vi "Axis-To-SIAM-direkt.vi"(7 "Extra Information":u32=255, 8 "error in (no error)":errorcluster, 10 "Position":dbl(slide)=1021459.0 scale=0.0..1000.0, 11 "Axis-Ring":T4=16777217 items=["255Axis"=16777217, "1-Axis"=17825793, "2-Axis"=18874369, "3-Axis"=19922945, "4-Axis"=20971521, "5-Axis"=22020097, "6-Axis"=23068673, "7-Axis"=24117249, "LED365"=2684354561, "LED385"=2685403137, "LED440"=2686451713, "LED470"=2687500289, "LED510"=2688548865, "LED540"=2689597441, "LED590"=2690646017, "LED640"=2691694593, "DurchR"=2701131777, "DurchG"=2702180353, "DurchB"=2703228929, "AF"=2704277505, "Laser0"=2717908993, "Laser1"=2718957569, "Laser2"=2720006145, "Laser3"=2721054721, "Servo0"=67108865, "Servo1"=68157441, "Servo2"=69206017, "Servo3"=70254593, "0-TMSI"=100663361, "1-TMSI"=101711937, "x-tmsi"=102760513, "y-tmsi"=103809089, "z-tmsi"=104857665, "orca1"=503316481, "orca2"=503316482, "orca3"=503316483, "orca4"=503316484, ""=0]) -> (0 "error out":errorcluster, 3 "Direct Commands":T6(array[cluster]) {"command" format="%x" items=["end_no_ticket"=4027514895, "end_ticket"=4027518991, "NoOp"=4026531840, "Read ticks"=4026535936, "Read ticks to var"=4026535938, "Read IP"=4043313152, "Read IP into var"=4043313154, "Set IP from var"=4043309059, "Set IP from var, relative"=4043313155, "branchRel_if_equal"=4043374849, "decrement_branchRel_if_equal"=4043374945, "decrement_branchRel_if_greaterequal"=4043375201, "decrement_branchRel_if_greaterequal_withTicket"=4043379297, "decrement_branchRel_if_smaller"=4043375457, "increment_branchRel_if_smaller"=4043375473, "readVar"=4060090368, "writeVar"=4060086273, "copyVar0_from_var1"=4060086275, "math_addToVariable"=4076863488, "math_addVToVariable"=4076863489, "math_subToVariable"=4076863490, "math_subVToVariable"=4076863491, "math_multToVariable"=4076863492, "math_multvToVariable"=4076863493, "math_divideToVariable"=4076863494, "math_divideVToVariable"=4076863495, "math_modToVariable"=4076863496, "math_modVToVariable"=4076863497, "logic_and"=4093640704, "logic_or"=4093640706, "logic_xor"=4093640708, "bitshift"=4093640712, "I2C-write"=335544337, "I2C-read"=335548433, "Cam-SPI-write"=3254779905, "UART0-VC-Baud-write"=469958673, "UART0-VC-Baud-read"=469962768, "UART0-VC-write"=469762065, "UART0-VC-write-Var"=469762067, "UART0-VC-read-availabe-bytes-to-var"=470355970, "UART0-VC-read-availabe-bytes"=470355984, "UART0-VC-read-skip-bytes"=469831681, "UART0-VC-read"=469766160, "UART0-VC-read-Var"=469766162, "UART1-TSM-Baud-write"=486735889, "UART1-TSM-Baud-read"=486739984, "UART1-TSM-write"=486539281, "UART1-TSM-write-Var"=486539283, "UART1-TSM-read-availabe-bytes-to-var"=487133186, "UART1-TSM-read-availabe-bytes"=487133200, "UART1-TSM-read-skip-bytes"=486604801, "UART1-TSM-read-skip-bytes"=486608897, "UART1-TSM-read"=486543376, "UART1-TSM-read-Var"=486543378, "UART2-Laser-Baud-write"=503513105, "UART2-Baud-read"=503517200, "UART2-write"=503316497, "UART2-write-Var"=503316499, "UART2-read-availabe-bytes-to-var"=503910402, "UART2-read-availabe-bytes"=503910416, "UART2-read-skip-bytes"=503386113, "UART2-read"=503320592, "UART2-read-Var"=503320594, "UART3-Baud-write"=520290321, "UART3-Baud-read"=520294416, "UART3-write"=520093713, "UART3-write-Var"=520093715, "UART3-read-availabe-bytes-to-var"=520687618, "UART3-read-availabe-bytes"=520687632, "UART3-read-skip-bytes"=520163329, "UART3-read"=520097808, "UART3-read-Var"=520097810, "IO-read_bank0"=3489665024, "IO-write_bank0"=3489660929, "IO-read_bank1"=3506442240, "IO-write_bank1"=3506438145, "DA0-0_LED365"=2684354561, "DA0-1_LED385"=2685403137, "DA0-2_LED440"=2686451713, "DA0-3_LED470"=2687500289, "DA0-4_LED510"=2688548865, "DA0-5_LED550"=2689597441, "DA0-6_LED590"=2690646017, "DA0-7_LED640"=2691694593, "DA1-0_LED-R"=2701131777, "DA1-1_LED-G"=2702180353, "DA1-2_LED-B"=2703228929, "DA1-3_LED-AF"=2704277505, "DA1-4"=2705326081, "DA1-5"=2706374657, "DA1-6"=2707423233, "DA1-7"=2708471809, "DA2-Laser0"=2717908993, "DA2-Laser1"=2718957569, "DA2-Laser2"=2720006145, "DA2-Laser3"=2721054721, "DA2-Laser4"=2722103297, "Analog-read_AD0-0"=2818576384, "Analog-read-store_AD0-0"=2818572290, "AF-Register-transfer r/w"=2835349505, "AF-Register-read"=2835353600, "AF-Register-read-to-var"=2835353602, "AF-Transfer-from-var"=2835349507, "IO-delay_bank0"=3489923073, "IO-delay_bank0_fromVar"=3489923075, "read_cam_clock"=3289124864, "store_cam_clock"=3289120770, "read_cam_phase"=3289190400, "store_cam_phase"=3289186306, "store_cam_phase-t"=3289190402, "r_cam1_NHS"=3254980608, "w_cam1_NHS"=3254976513, "r_cam1_NVS"=3255046144, "w_cam1_NVS"=3255042049, "r_cam1_npx"=3255111680, "w_cam1_npx"=3255107585, "r_cam1_npy"=3255177216, "w_cam1_npy"=3255173121, "r_cam1_xhswait"=3255439360, "w_cam1_xhswait"=3255435265, "r_cam1_xvs_wait"=3255504896, "w_cam1_xvs_wait"=3255500801, "r_cam1_framcounter"=3255570432, "r_cam1_line"=3255635968, "r_cam1_xhs-counter"=3255701504, "r_cam2_NHS"=3271757824, "w_cam2_NHS"=3271753729, "r_cam2_NVS"=3271823360, "w_cam2_NVS"=3271819265, "r_cam2_npx"=3271888896, "w_cam2_npx"=3271884801, "r_cam2_npy"=3271954432, "w_cam2_npy"=3271950337, "r_cam2_xvs_wait"=3272282112, "w_cam2_xvs_wait"=3272278017, "r_cam2_framcounter"=3272347648, "r_cam2_line"=3272413184, "r_cam2_xhs-counter"=3272478720, "start TMSI"=102694919, "set_1Galvo"=101712113, "set_x-Galvo"=102760689, "set_y-Galvo"=103809265, "set_z-Fokus"=104857841, "set_1Galvo_position-only"=101711937, "set_x-Galvo_position-only"=102760513, "set_y-Galvo_position-only"=103809089, "set_z-Fokus_position-only"=104857665, "set_x-Galvo_position-only_ticket"=102764609, "set_y-Galvo_position-only_ticket"=103813185, "set_z-Fokus_position-only_ticket"=104861761, "set_1Galvo_relativ-only"=101712001, "set_x-Galvo_relativ-only"=102760577, "set_y-Galvo_relativ-only"=103809153, "set_z-Fokus_relativ-only"=104857729, "set_1Galvo_speed-only"=101711905, "set_x-Galvo_speed-only"=102760481, "set_y-Galvo_speed-only"=103809057, "set_z-Fokus_speed-only"=104857633, "set_1Galvo_acc-only"=101711889, "set_x-Galvo_acc-only"=102760465, "set_y-Galvo_acc-only"=103809041, "set_z-Fokus_acc-only"=104857617, "read_1Galvo_ticket"=101716032, "read_x-Galvo_ticket"=102764608, "read_y-Galvo_ticket"=103813184, "read_z-Focus_ticket"=104861760, "x-Galvo_pos_fromVar"=102760515, "y-Galvo_pos_fromVar"=103809091, "z-Focus_pos_fromVar"=104857667, "Servo0"=67108865, "Servo0-enable"=68091911, "Servo0-disable"=68091919, "Servo1"=68157441, "Servo1-enable"=69140487, "Servo1-disable"=69140495, "Servo2-enable"=70189063, "Servo2"=69206017, "Servo3-enable"=71237639, "Servo3"=70254593, "x-ssi-init"=202309639, "x-ssi-disable"=202309647, "x-ssi-Bits"=201523201, "x-ssi-Read"=201330688, "x-ssi-ReadToVar"=201326594, "x-ssi-ReadToVar-ticket"=201330690, "y-ssi-init"=203358215, "y-ssi-disable"=203358223, "y-ssi-Bits"=202571777, "y-ssi-Read"=202379264, "y-ssi-ReadToVar"=202375170, "y-ssi-ReadToVat-ticket"=202379266]; "P5-ticket" format="%.0x"; "Delay 10µs" format="%.0x"; "P0" format="%.0x"; "P1" format="%.0x"})   [LabVIEW 2011]
uses:
  SIAM_command.ctl
  SIAM-axis.ctl
panel:
  out "TSM cluster":T1
  out "orca string":string
  out "Motor":T2(ring)
  in  "ScaleConst":T3(array[cluster])=[{"Axis-Ring"=104857665, "Scale"=-128000.0, "Offset"=-1000000.0, "HW min"=-3000000.0, "HW max"=0.0, "max a"=inf, "max v"=inf, "units"="µm"}, {"Axis-Ring"=102760513, "Scale"=1.0, "Offset"=-4000.0, "HW min"=-32000.0, "HW max"=32000.0, "max a"=5.0, "max v"=inf, "units"="c"}, {"Axis-Ring"=101711937, "Scale"=1.0, "Offset"=0.0, "HW min"=-32000.0, "HW max"=32000.0, "max a"=0.02, "max v"=inf, "units"="c"}, {"Axis-Ring"=16777217, "Scale"=51200.0, "Offset"=100.0, "HW min"=0.0, "HW max"=5500000.0, "max a"=inf, "max v"=20.0, "units"="mm"}, {"Axis-Ring"=17825793, "Scale"=51200.0, "Offset"=100.0, "HW min"=0.0, "HW max"=3700000.0, "max a"=inf, "max v"=20.0, "units"="mm"}, {"Axis-Ring"=19922945, "Scale"=153600.0, "Offset"=146600.0, "HW min"=0.0, "HW max"=614400.0, "max a"=inf, "max v"=inf, "units"="Pos"}, {"Axis-Ring"=20971521, "Scale"=25000.1, "Offset"=641.0, "HW min"=0.0, "HW max"=124721.0, "max a"=inf, "max v"=inf, "units"="Pos"}, {"Axis-Ring"=22020097, "Scale"=1.0, "Offset"=0.0, "HW min"=0.0, "HW max"=51200.0, "max a"=inf, "max v"=inf, "units"="counts"}, {"Axis-Ring"=23068673, "Scale"=10240.0, "Offset"=0.0, "HW min"=0.0, "HW max"=51200.0, "max a"=inf, "max v"=inf, "units"="Pos"}, {"Axis-Ring"=24117249, "Scale"=1.0, "Offset"=0.0, "HW min"=0.0, "HW max"=51200.0, "max a"=inf, "max v"=inf, "units"="counts"}, {"Axis-Ring"=2684354561, "Scale"=1.0, "Offset"=0.0, "HW min"=0.0, "HW max"=65636.0, "max a"=inf, "max v"=inf, "units"="counts"}, {"Axis-Ring"=2685403137, "Scale"=1.0, "Offset"=0.0, "HW min"=0.0, "HW max"=65636.0, "max a"=inf, "max v"=inf, "units"="counts"}, {"Axis-Ring"=2686451713, "Scale"=1.0, "Offset"=0.0, "HW min"=0.0, "HW max"=65636.0, "max a"=inf, "max v"=inf, "units"="counts"}, {"Axis-Ring"=2687500289, "Scale"=1.0, "Offset"=0.0, "HW min"=0.0, "HW max"=65636.0, "max a"=inf, "max v"=inf, "units"="counts"}, {"Axis-Ring"=2688548865, "Scale"=1.0, "Offset"=0.0, "HW min"=0.0, "HW max"=65636.0, "max a"=inf, "max v"=inf, "units"="counts"}, {"Axis-Ring"=2689597441, "Scale"=1.0, "Offset"=1.0, "HW min"=0.0, "HW max"=65636.0, "max a"=inf, "max v"=inf, "units"="counts"}, {"Axis-Ring"=2690646017, "Scale"=1.0, "Offset"=1.0, "HW min"=0.0, "HW max"=65636.0, "max a"=inf, "max v"=inf, "units"="counts"}, {"Axis-Ring"=2691694593, "Scale"=1.0, "Offset"=1.0, "HW min"=0.0, "HW max"=65636.0, "max a"=inf, "max v"=inf, "units"="counts"}, {"Axis-Ring"=2701131777, "Scale"=1.0, "Offset"=1.0, "HW min"=0.0, "HW max"=65636.0, "max a"=inf, "max v"=inf, "units"="counts"}, {"Axis-Ring"=2702180353, "Scale"=1.0, "Offset"=1.0, "HW min"=0.0, "HW max"=65636.0, "max a"=inf, "max v"=inf, "units"="counts"}, {"Axis-Ring"=2703228929, "Scale"=1.0, "Offset"=1.0, "HW min"=0.0, "HW max"=65636.0, "max a"=inf, "max v"=inf, "units"="counts"}, {"Axis-Ring"=2704277505, "Scale"=1.0, "Offset"=1.0, "HW min"=0.0, "HW max"=65636.0, "max a"=inf, "max v"=inf, "units"="counts"}, {"Axis-Ring"=2717908993, "Scale"=1.0, "Offset"=1.0, "HW min"=0.0, "HW max"=65636.0, "max a"=inf, "max v"=inf, "units"="counts"}, {"Axis-Ring"=2718957569, "Scale"=1.0, "Offset"=1.0, "HW min"=0.0, "HW max"=65636.0, "max a"=inf, "max v"=inf, "units"="counts"}, {"Axis-Ring"=2720006145, "Scale"=1.0, "Offset"=1.0, "HW min"=0.0, "HW max"=65636.0, "max a"=inf, "max v"=inf, "units"="counts"}, {"Axis-Ring"=2721054721, "Scale"=1.0, "Offset"=1.0, "HW min"=0.0, "HW max"=65636.0, "max a"=inf, "max v"=inf, "units"="counts"}, {"Axis-Ring"=67108865, "Scale"=1.0, "Offset"=1.0, "HW min"=100000.0, "HW max"=200000.0, "max a"=inf, "max v"=inf, "units"="counts"}, {"Axis-Ring"=68157441, "Scale"=1.0, "Offset"=1.0, "HW min"=100000.0, "HW max"=200000.0, "max a"=inf, "max v"=inf, "units"="counts"}] {"Axis-Ring" items=["Galvo1"=101711937, "x-Galvo"=102760513, "z-Fokus"=104857665, "X-Axis"=16777217, "Y-Axis"=17825793, "Obj"=19922945, "Filter"=20971521, "Trans"=22020097, "FRET"=23068673, "SI"=24117249, "LED385"=2685403137, "LED440"=2686451713, "LED470"=2687500289, "LED510"=2688548865, "LED540"=2689597441, "LED590"=2690646017, "LED640"=2691694593, "DurchR"=2701131777, "DurchG"=2702180353, "DurchB"=2703228929, "AF"=2704277505, "Laser0"=2717908993, "Laser1"=2718957569, "Laser2"=2720006145, "Laser3"=2721054721, "Servo0"=67108865, "Servo1"=68157441]}
  # "e.g. Technosoft conneted to UART"
  # "UART geht so leider nicht, direktbefehle könne keine Pause> read zu früh..."
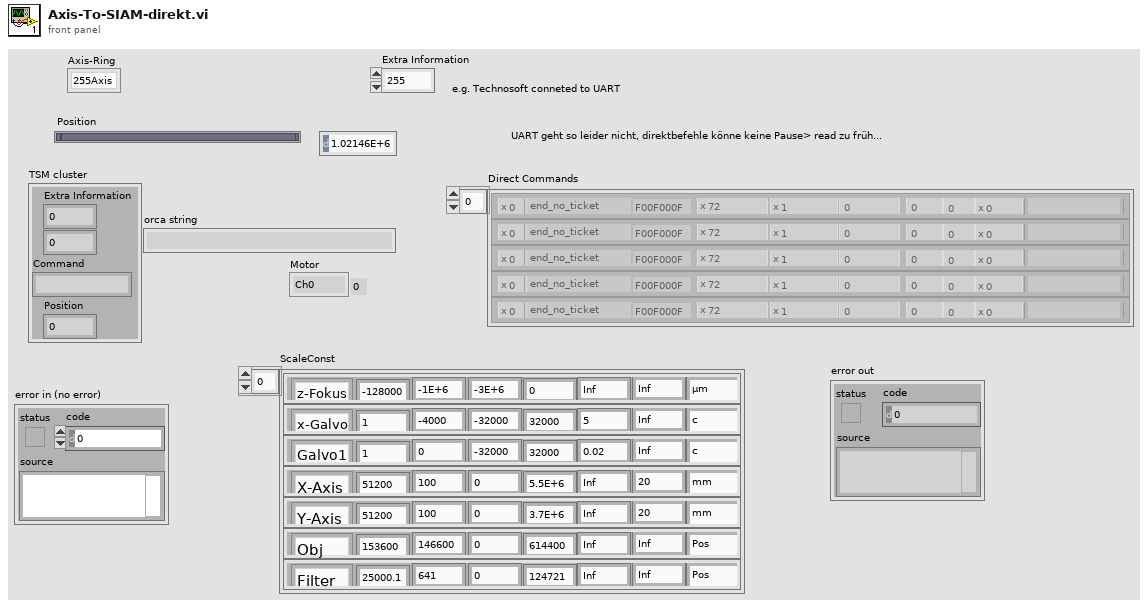
[diagram p1: front panel]
types:
  T1 = cluster{"Extra Information":u32, i32, "Command":string, "Position":dbl}
  T2 = enum8{"Ch0", "Ch1", "x-Galvo", "y-Galvo", "z-Focus"}
  T3 = cluster{"Axis-Ring":u32, "Scale":dbl, "Offset":dbl, "HW min":dbl, "HW max":dbl, "max a":dbl, "max v":dbl, "units":string}[]
  T4 = typedef "SIAM-axis.ctl" = u32
  T5 = typedef "SIAM_command.ctl" = u32
  T6 = cluster{"Delay 10µs":u32, "command":T5, "P0":i32, "P1":i32, "P2":i32, "P3":i32, "P4":i32, "P5-ticket":i32, "comment":string}[]
  T7 = cluster{"rel 10µs":u32, "Device":T5, "data0":i32, "data1":i32, "data2":i32, "data3":i32, "data4":i32, "data5":i32, string}
  T8 = cluster{"rel 10µs":u32, "Device":T5, "data0":i32, "data1":i32, "data2":i32, "data3":i32, "data4":i32, "data5":i32, string}[]
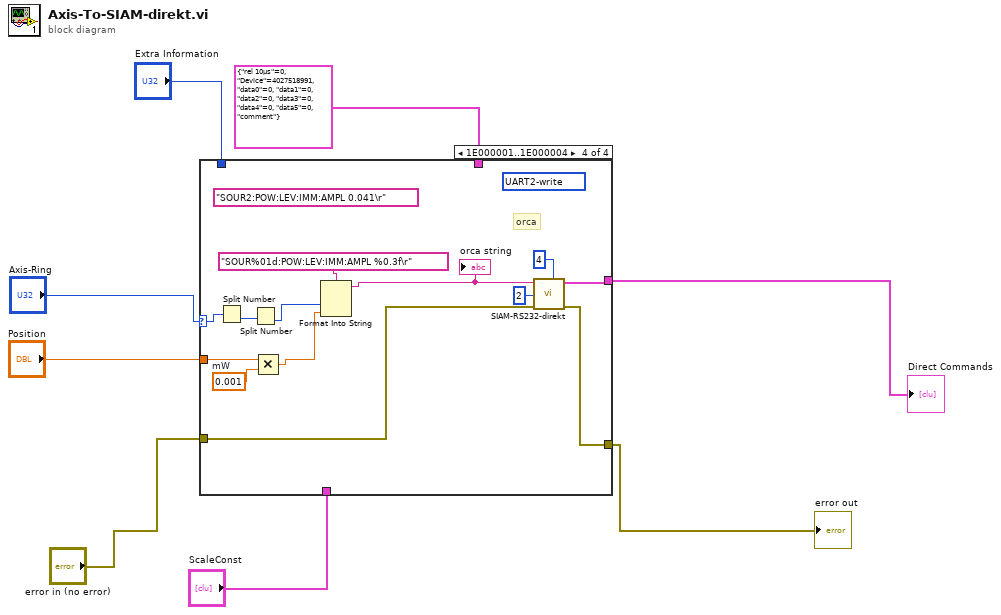
[diagram p0: block diagram]
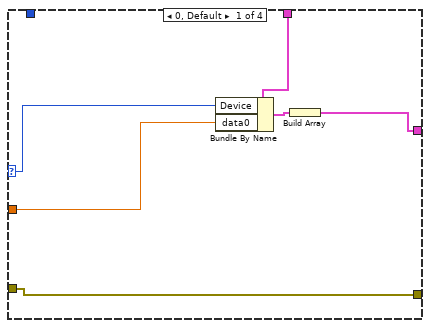
[diagram p2: hidden frame]
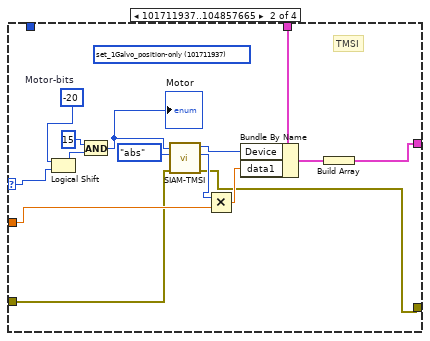
[diagram p3: hidden frame]
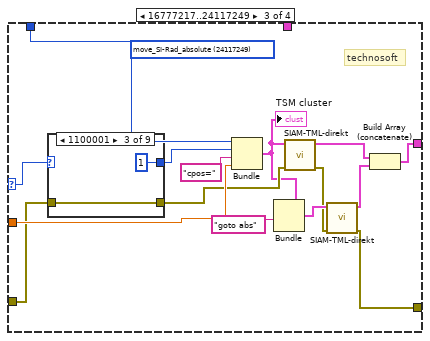
[diagram p4: hidden frame]
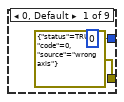
[diagram p5: hidden frame]
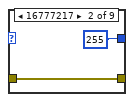
[diagram p6: hidden frame]
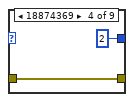
[diagram p7: hidden frame]
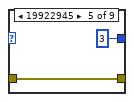
[diagram p8: hidden frame]
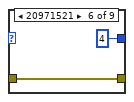
[diagram p9: hidden frame]
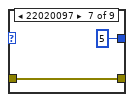
[diagram p10: hidden frame]
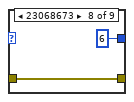
[diagram p11: hidden frame]
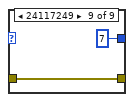
[diagram p12: hidden frame]
diagram:
  n1 = case shown="1E000001..1E000004" "Axis-Ring" {
    selector: "Axis-Ring" -> [w14 w19 w34 w71]
    tunnel: [w10 w22 w39 w75] -> w5
    tunnel: "Position" -> [w13 w25 w43 w68]
    tunnel: T7 {"rel 10µs"=0, "Device"=4027518991, "data0"=0, "data1"=0, "data2"=0, "data3"=0, "data4"=0, "data5"=0, "comment"} ("output cluster") -> [w11 w26 _ _]
    tunnel: "ScaleConst" -> [_ _ _ _]
    tunnel: "error in (no error)" -> [w9 w21 w32 w73]
    tunnel: [w9 w20 w37 w72] -> w2
    tunnel: "Extra Information" -> [_ _ w35 _]
    frame 0, Default {
      n2 = Bundle By Name(cluster=w11, "Device"=w14, "data0"=w13) -> (w12:T7)
      n3 = Build Array(w12) -> (w10:T8)
    }
    frame 101711937..104857665 {
      w18 = i8 -20  # Motor-bits
      (unwired) T5 101711937 items=["read_x-Motor_status_ticket"=17305600, "init_x-Motor"=17760263, "read_x-Motor_absolute_ticket"=16781312, "move_x-Motor_absolute"=16777217, "move_x-Motor_relative"=16842753, "read_x-Motor_speed"=16977920, "set_x-Motor_speed"=16973825, "read_y-Motor_status_ticket"=18354176, "init_y-Motor"=18808839, "read_y-Motor_absolute_ticket"=17829888, "move_y-Motor_absolute"=17825793, "move_y-Motor_relative"=17891329, "read_y-Motor_speed"=18026496, "set_y-Motor_speed"=18022401, "read_z-Motor_status_ticket"=19402752, "init_z-Motor"=19857415, "stop_z-Motor"=19857423, "start_z-Motor"=19857422, "read_z-Motor_absolute_ticket"=18878464, "move_z-Motor_absolute"=18874369, "move_z-Motor_relative"=18939905, "read_Objective_status_ticket"=20451328, "init_Objective"=20905991, "read_Objective_absolute_ticket"=19927040, "move_Objective_absolute"=19922945, "move_Objective_relative"=19988481, "read_Objective-Motor_speed"=20123648, "set_Objective-Motor_speed"=20119553, "read_Filter_status_ticket"=21499904, "init_Filter"=21954567, "read_Filter_absolute_ticket"=20975616, "move_Filter_absolute"=20971521, "move_Filter_relative"=21037057, "read_Filter-Motor_speed"=21172224, "set_Filter-Motor_speed"=21168129, "read_Trans-Rad_status_ticket"=22548480, "init_Trans-Rad"=23003143, "read_Trans-Rad_absolute_ticket"=22024192, "move_Trans-Rad_absolute"=22020097, "move_Trans-Rad_relative"=22085633, "read_Trans-Motor_speed"=22220800, "set_Trans-Motor_speed"=22216705, "read_FRET_status_ticket"=23597056, "init_FRET"=24051719, "read_FRET_absolute_ticket"=23072768, "move_FRET_absolute"=23068673, "move_FRET_relative"=23134209, "read_FRET-Motor_speed"=23269376, "set_FRET-Motor_speed"=23265281, "read_SI-Rad_status_ticket"=24645632, "init_SI-Rad"=25100295, "read_SI-Rad_absolute_ticket"=24121344, "move_SI-Rad_absolute"=24117249, "move_SI-Rad_relative"=24182785, "read_SI-Rad_speed"=24317952, "set_SI-Rad_speed"=24313857, "I2C-write"=335544337, "I2C-read"=335548433, "UART0-VC-Baud-write"=469958673, "UART0-VC-Baud-read"=469962768, "UART0-VC-write"=469762065, "UART0-VC-write-Var"=469762067, "UART0-VC-read"=469766160, "UART0-VC-read-Var"=469766162, "UART1-TSM-Baud-read"=486739984, "UART1-TSM-write"=486539281, "UART1-TSM-write-ticket"=486543377, "UART1-TSM-write-var-binary"=486539283, "UART1-TSM-write-var-binary-ticket"=486543379, "UART1-TSM-read"=486543376, "UART1-TSM-read-var-binary"=486543378, "UART2-write"=503316497, "UART2-read"=503320592, "USB-UART0-write"=536870929, "USB-UART0-read"=536875024, "USB-UART0-Float-Bitschift"=537133073, "USB-UART0-read-Float"=536875234, "USB-UART0-write-Float"=536871139, "USB-UART0-read-Float"=536875250, "USB-UART0-write-Float"=536871155, "end_no_ticket"=4027514895, "end_ticket"=4027518991, "NoOp"=4060086272, "IO-read_bank0"=3489665024, "IO-write_bank0"=3489660929, "IO-read_bank1"=3506442240, "IO-write_bank1"=3506438145, "DA0-0_LED365"=2684354561, "DA0-1_LED385"=2685403137, "DA0-2_LED440"=2686451713, "DA0-3_LED470"=2687500289, "DA0-4_LED510"=2688548865, "DA0-5_LED550"=2689597441, "DA0-6_LED590"=2690646017, "DA0-7_LED640"=2691694593, "DA1-0_LED-R"=2701131777, "DA1-1_LED-G"=2702180353, "DA1-2_LED-B"=2703228929, "DA1-3_LED-AF"=2704277505, "DA1-4"=2705326081, "DA1-5"=2706374657, "DA1-6"=2707423233, "DA1-7"=2708471809, "DA2-Laser0"=2717908993, "DA2-Laser1"=2718957569, "DA2-Laser2"=2720006145, "DA2-Laser3"=2721054721, "DA2-Laser4"=2722103297, "Analog-read_AD0-0"=2818576384, "Analog-read-store_AD0-0"=2818572290, "IO-delay_bank0"=3489923073, "IO-delay_bank0_fromVar"=3489923075, "read_cam_clock"=3289124864, "store_cam_clock"=3289120770, "read_cam_phase"=3289190400, "store_cam_phase"=3289186306, "store_cam_phase-t"=3289190402, "Read ticks"=4026535936, "Read ticks to var"=4026535938, "Read IP"=4043313152, "Read IP into var"=4043313154, "Set IP from var"=4043309059, "Set IP from var, relative"=4043313155, "decrement_branchRel_if_equal"=4043374945, "decrement_branchRel_if_greaterequal"=4043375201, "decrement_branchRel_if_greaterequal_withTicket"=4043379297, "decrement_branchRel_if_smaller"=4043375457, "increment_branchRel_if_smaller"=4043375473, "readVar"=4060090368, "writeVar"=4060086273, "copyVar0_from_var1"=4060086275, "math_addToVariable"=4076863488, "math_addVToVariable"=4076863489, "math_subToVariable"=4076863490, "math_subVToVariable"=4076863491, "math_multToVariable"=4076863492, "math_multvToVariable"=4076863493, "math_divideToVariable"=4076863494, "math_divideVToVariable"=4076863495, "math_modToVariable"=4076863496, "math_modVToVariable"=4076863497, "logic_and"=4093640704, "logic_or"=4093640706, "logic_xor"=4093640708, "bitshift"=4093640712, "set_1Galvo"=101712113, "set_x-Galvo"=102760689, "set_y-Galvo"=103809265, "set_z-Fokus"=104857841, "set_1Galvo_position-only"=101711937, "set_x-Galvo_position-only"=102760513, "set_y-Galvo_position-only"=103809089, "set_z-Fokus_position-only"=104857665, "set_x-Galvo_position-only_ticket"=102764609, "set_y-Galvo_position-only_ticket"=103813185, "set_z-Fokus_position-only_ticket"=104861761, "set_1Galvo_relativ-only"=101712001, "set_x-Galvo_relativ-only"=102760577, "set_y-Galvo_relativ-only"=103809153, "set_z-Fokus_relativ-only"=104857729, "set_1Galvo_speed-only"=101711905, "set_x-Galvo_speed-only"=102760481, "set_y-Galvo_speed-only"=103809057, "set_z-Fokus_speed-only"=104857633, "set_1Galvo_acc-only"=101711889, "set_x-Galvo_acc-only"=102760465, "set_y-Galvo_acc-only"=103809041, "set_z-Fokus_acc-only"=104857617, "read_1Galvo_ticket"=101716032, "read_x-Galvo_ticket"=102764608, "read_y-Galvo_ticket"=103813184, "read_z-Focus_ticket"=104861760, "x-Galvo_pos_fromVar"=102760515, "y-Galvo_pos_fromVar"=103809091, "z-Focus_pos_fromVar"=104857667, "Servo0"=67108865, "Servo0-enable"=68091911, "Servo0-disable"=68091919, "Servo1"=68157441, "Servo1-enable"=69140487, "Servo1-disable"=69140495, "Servo2-enable"=70189063, "Servo2"=69206017, "Servo3-enable"=71237639, "Servo3"=70254593, "x-ssi-init"=202309639, "x-ssi-disable"=202309647, "x-ssi-Bits"=201523201, "x-ssi-Read"=201330688, "x-ssi-ReadToVar"=201326594, "x-ssi-ReadToVar-ticket"=201330690, "y-ssi-init"=203358215, "y-ssi-disable"=203358223, "y-ssi-Bits"=202571777, "y-ssi-Read"=202379264, "y-ssi-ReadToVar"=202375170, "y-ssi-ReadToVat-ticket"=202379266] ("command")
      # "TMSI"
      n4 = Logical Shift(y=w18, x=w19) -> (x << y=w17:T4)
      n5 = And(x=u32 15 ("mask"), y=w17) -> (x .and. y?=w15:T4)
      "Motor" <- w15
      n6 = call "SIAM-TMSI.vi"("error in (no error)"=w21, "Type"=enum8{"acc", "vel", "abs", "offset"}."abs", "Motor"=w15) -> ("error out"=w20:errorcluster, "Resolution-Factor"=w24:i32, "command"=w28:T5)  [unwired: 5 in, 1 out]
      n7 = Multiply(x=w24, y=w25) -> (x*y=w23:dbl)
      n8 = Bundle By Name(cluster=w26, "Device"=w28, "data1"=w23) -> (w27:T7)
      n9 = Build Array(w27) -> (w22:T8)
    }
    frame 16777217..24117249 {
      (unwired) T5 24117249 items=["read_x-Motor_status_ticket"=17305600, "init_x-Motor"=17760263, "read_x-Motor_absolute_ticket"=16781312, "move_x-Motor_absolute"=16777217, "move_x-Motor_relative"=16842753, "read_x-Motor_speed"=16977920, "set_x-Motor_speed"=16973825, "read_y-Motor_status_ticket"=18354176, "init_y-Motor"=18808839, "read_y-Motor_absolute_ticket"=17829888, "move_y-Motor_absolute"=17825793, "move_y-Motor_relative"=17891329, "read_y-Motor_speed"=18026496, "set_y-Motor_speed"=18022401, "read_z-Motor_status_ticket"=19402752, "init_z-Motor"=19857415, "stop_z-Motor"=19857423, "start_z-Motor"=19857422, "read_z-Motor_absolute_ticket"=18878464, "move_z-Motor_absolute"=18874369, "move_z-Motor_relative"=18939905, "read_Objective_status_ticket"=20451328, "init_Objective"=20905991, "read_Objective_absolute_ticket"=19927040, "move_Objective_absolute"=19922945, "move_Objective_relative"=19988481, "read_Objective-Motor_speed"=20123648, "set_Objective-Motor_speed"=20119553, "read_Filter_status_ticket"=21499904, "init_Filter"=21954567, "read_Filter_absolute_ticket"=20975616, "move_Filter_absolute"=20971521, "move_Filter_relative"=21037057, "read_Filter-Motor_speed"=21172224, "set_Filter-Motor_speed"=21168129, "read_Trans-Rad_status_ticket"=22548480, "init_Trans-Rad"=23003143, "read_Trans-Rad_absolute_ticket"=22024192, "move_Trans-Rad_absolute"=22020097, "move_Trans-Rad_relative"=22085633, "read_Trans-Motor_speed"=22220800, "set_Trans-Motor_speed"=22216705, "read_FRET_status_ticket"=23597056, "init_FRET"=24051719, "read_FRET_absolute_ticket"=23072768, "move_FRET_absolute"=23068673, "move_FRET_relative"=23134209, "read_FRET-Motor_speed"=23269376, "set_FRET-Motor_speed"=23265281, "read_SI-Rad_status_ticket"=24645632, "init_SI-Rad"=25100295, "read_SI-Rad_absolute_ticket"=24121344, "move_SI-Rad_absolute"=24117249, "move_SI-Rad_relative"=24182785, "read_SI-Rad_speed"=24317952, "set_SI-Rad_speed"=24313857, "I2C-write"=335544337, "I2C-read"=335548433, "UART0-VC-Baud-write"=469958673, "UART0-VC-Baud-read"=469962768, "UART0-VC-write"=469762065, "UART0-VC-write-Var"=469762067, "UART0-VC-read"=469766160, "UART0-VC-read-Var"=469766162, "UART1-TSM-Baud-read"=486739984, "UART1-TSM-write"=486539281, "UART1-TSM-write-ticket"=486543377, "UART1-TSM-write-var-binary"=486539283, "UART1-TSM-write-var-binary-ticket"=486543379, "UART1-TSM-read"=486543376, "UART1-TSM-read-var-binary"=486543378, "UART2-write"=503316497, "UART2-read"=503320592, "USB-UART0-write"=536870929, "USB-UART0-read"=536875024, "USB-UART0-Float-Bitschift"=537133073, "USB-UART0-read-Float"=536875234, "USB-UART0-write-Float"=536871139, "USB-UART0-read-Float"=536875250, "USB-UART0-write-Float"=536871155, "end_no_ticket"=4027514895, "end_ticket"=4027518991, "NoOp"=4060086272, "IO-read_bank0"=3489665024, "IO-write_bank0"=3489660929, "IO-read_bank1"=3506442240, "IO-write_bank1"=3506438145, "DA0-0_LED365"=2684354561, "DA0-1_LED385"=2685403137, "DA0-2_LED440"=2686451713, "DA0-3_LED470"=2687500289, "DA0-4_LED510"=2688548865, "DA0-5_LED550"=2689597441, "DA0-6_LED590"=2690646017, "DA0-7_LED640"=2691694593, "DA1-0_LED-R"=2701131777, "DA1-1_LED-G"=2702180353, "DA1-2_LED-B"=2703228929, "DA1-3_LED-AF"=2704277505, "DA1-4"=2705326081, "DA1-5"=2706374657, "DA1-6"=2707423233, "DA1-7"=2708471809, "DA2-Laser0"=2717908993, "DA2-Laser1"=2718957569, "DA2-Laser2"=2720006145, "DA2-Laser3"=2721054721, "DA2-Laser4"=2722103297, "Analog-read_AD0-0"=2818576384, "Analog-read-store_AD0-0"=2818572290, "IO-delay_bank0"=3489923073, "IO-delay_bank0_fromVar"=3489923075, "read_cam_clock"=3289124864, "store_cam_clock"=3289120770, "read_cam_phase"=3289190400, "store_cam_phase"=3289186306, "store_cam_phase-t"=3289190402, "Read ticks"=4026535936, "Read ticks to var"=4026535938, "Read IP"=4043313152, "Read IP into var"=4043313154, "Set IP from var"=4043309059, "Set IP from var, relative"=4043313155, "decrement_branchRel_if_equal"=4043374945, "decrement_branchRel_if_greaterequal"=4043375201, "decrement_branchRel_if_greaterequal_withTicket"=4043379297, "decrement_branchRel_if_smaller"=4043375457, "increment_branchRel_if_smaller"=4043375473, "readVar"=4060090368, "writeVar"=4060086273, "copyVar0_from_var1"=4060086275, "math_addToVariable"=4076863488, "math_addVToVariable"=4076863489, "math_subToVariable"=4076863490, "math_subVToVariable"=4076863491, "math_multToVariable"=4076863492, "math_multvToVariable"=4076863493, "math_divideToVariable"=4076863494, "math_divideVToVariable"=4076863495, "math_modToVariable"=4076863496, "math_modVToVariable"=4076863497, "logic_and"=4093640704, "logic_or"=4093640706, "logic_xor"=4093640708, "bitshift"=4093640712, "set_1Galvo"=101712113, "set_x-Galvo"=102760689, "set_y-Galvo"=103809265, "set_z-Fokus"=104857841, "set_1Galvo_position-only"=101711937, "set_x-Galvo_position-only"=102760513, "set_y-Galvo_position-only"=103809089, "set_z-Fokus_position-only"=104857665, "set_x-Galvo_position-only_ticket"=102764609, "set_y-Galvo_position-only_ticket"=103813185, "set_z-Fokus_position-only_ticket"=104861761, "set_1Galvo_relativ-only"=101712001, "set_x-Galvo_relativ-only"=102760577, "set_y-Galvo_relativ-only"=103809153, "set_z-Fokus_relativ-only"=104857729, "set_1Galvo_speed-only"=101711905, "set_x-Galvo_speed-only"=102760481, "set_y-Galvo_speed-only"=103809057, "set_z-Fokus_speed-only"=104857633, "set_1Galvo_acc-only"=101711889, "set_x-Galvo_acc-only"=102760465, "set_y-Galvo_acc-only"=103809041, "set_z-Fokus_acc-only"=104857617, "read_1Galvo_ticket"=101716032, "read_x-Galvo_ticket"=102764608, "read_y-Galvo_ticket"=103813184, "read_z-Focus_ticket"=104861760, "x-Galvo_pos_fromVar"=102760515, "y-Galvo_pos_fromVar"=103809091, "z-Focus_pos_fromVar"=104857667, "Servo0"=67108865, "Servo0-enable"=68091911, "Servo0-disable"=68091919, "Servo1"=68157441, "Servo1-enable"=69140487, "Servo1-disable"=69140495, "Servo2-enable"=70189063, "Servo2"=69206017, "Servo3-enable"=71237639, "Servo3"=70254593, "x-ssi-init"=202309639, "x-ssi-disable"=202309647, "x-ssi-Bits"=201523201, "x-ssi-Read"=201330688, "x-ssi-ReadToVar"=201326594, "x-ssi-ReadToVar-ticket"=201330690, "y-ssi-init"=203358215, "y-ssi-disable"=203358223, "y-ssi-Bits"=202571777, "y-ssi-Read"=202379264, "y-ssi-ReadToVar"=202375170, "y-ssi-ReadToVat-ticket"=202379266] ("command")
      # "technosoft"
      n10 = case shown="1100001" w34 {
        tunnel: [0 255 1 2 3 4 5 6 7] -> w33
        tunnel: w32 -> [_ w47 w49 w51 w53 w55 w57 w59 w61]
        tunnel: [errorcluster {"status"=TRUE, "code"=0, "source"="wrong axis"} ("error in (no error)") w47 w49 w51 w53 w55 w57 w59 w61] -> w31
        frame 0, Default {
        }
        frame 16777217 {
        }
        frame 17825793 {
        }
        frame 18874369 {
        }
        frame 19922945 {
        }
        frame 20971521 {
        }
        frame 22020097 {
        }
        frame 23068673 {
        }
        frame 24117249 {
        }
      }
      n11 = Bundle("Extra Information"=w35, w33, "Command"="cpos=", "Position"=w43) -> (w30:T1)  [unwired: 1 in]
      "TSM cluster" <- w30
      n12 = Bundle(cluster=w30, "Command"="goto abs") -> (w42:T1)  [unwired: 3 in]
      n13 = call "SIAM-TML-direkt.vi"("error in (no error)"=w31, "TSM"=w30) -> ("error out"=w36:errorcluster, "Array"=w40:T6)  [unwired: 6 in, 2 out]
      n14 = call "SIAM-TML-direkt.vi"("error in (no error)"=w36, "TSM"=w42) -> ("error out"=w37:errorcluster, "Array"=w38:T6)  [unwired: 6 in, 2 out]
      n15 = Build Array (concatenate)(w40, w38) -> (w39:T6)
    }
    frame 503316481..503316484 {
      w66 = 0.001  # mW
      (unwired) "SOUR2:POW:LEV:IMM:AMPL 0.041\r"
      (unwired) T5 503316497 items=["read_x-Motor_status_ticket"=17305600, "init_x-Motor"=17760263, "read_x-Motor_absolute_ticket"=16781312, "move_x-Motor_absolute"=16777217, "move_x-Motor_relative"=16842753, "read_x-Motor_speed"=16977920, "set_x-Motor_speed"=16973825, "read_y-Motor_status_ticket"=18354176, "init_y-Motor"=18808839, "read_y-Motor_absolute_ticket"=17829888, "move_y-Motor_absolute"=17825793, "move_y-Motor_relative"=17891329, "read_y-Motor_speed"=18026496, "set_y-Motor_speed"=18022401, "read_z-Motor_status_ticket"=19402752, "init_z-Motor"=19857415, "stop_z-Motor"=19857423, "start_z-Motor"=19857422, "read_z-Motor_absolute_ticket"=18878464, "move_z-Motor_absolute"=18874369, "move_z-Motor_relative"=18939905, "read_Objective_status_ticket"=20451328, "init_Objective"=20905991, "read_Objective_absolute_ticket"=19927040, "move_Objective_absolute"=19922945, "move_Objective_relative"=19988481, "read_Objective-Motor_speed"=20123648, "set_Objective-Motor_speed"=20119553, "read_Filter_status_ticket"=21499904, "init_Filter"=21954567, "read_Filter_absolute_ticket"=20975616, "move_Filter_absolute"=20971521, "move_Filter_relative"=21037057, "read_Filter-Motor_speed"=21172224, "set_Filter-Motor_speed"=21168129, "read_Trans-Rad_status_ticket"=22548480, "init_Trans-Rad"=23003143, "read_Trans-Rad_absolute_ticket"=22024192, "move_Trans-Rad_absolute"=22020097, "move_Trans-Rad_relative"=22085633, "read_Trans-Motor_speed"=22220800, "set_Trans-Motor_speed"=22216705, "read_FRET_status_ticket"=23597056, "init_FRET"=24051719, "read_FRET_absolute_ticket"=23072768, "move_FRET_absolute"=23068673, "move_FRET_relative"=23134209, "read_FRET-Motor_speed"=23269376, "set_FRET-Motor_speed"=23265281, "read_SI-Rad_status_ticket"=24645632, "init_SI-Rad"=25100295, "read_SI-Rad_absolute_ticket"=24121344, "move_SI-Rad_absolute"=24117249, "move_SI-Rad_relative"=24182785, "read_SI-Rad_speed"=24317952, "set_SI-Rad_speed"=24313857, "I2C-write"=335544337, "I2C-read"=335548433, "UART0-VC-Baud-write"=469958673, "UART0-VC-Baud-read"=469962768, "UART0-VC-write"=469762065, "UART0-VC-write-Var"=469762067, "UART0-VC-read"=469766160, "UART0-VC-read-Var"=469766162, "UART1-TSM-Baud-read"=486739984, "UART1-TSM-write"=486539281, "UART1-TSM-write-ticket"=486543377, "UART1-TSM-write-var-binary"=486539283, "UART1-TSM-write-var-binary-ticket"=486543379, "UART1-TSM-read"=486543376, "UART1-TSM-read-var-binary"=486543378, "UART2-write"=503316497, "UART2-read"=503320592, "USB-UART0-write"=536870929, "USB-UART0-read"=536875024, "USB-UART0-Float-Bitschift"=537133073, "USB-UART0-read-Float"=536875234, "USB-UART0-write-Float"=536871139, "USB-UART0-read-Float"=536875250, "USB-UART0-write-Float"=536871155, "end_no_ticket"=4027514895, "end_ticket"=4027518991, "NoOp"=4060086272, "IO-read_bank0"=3489665024, "IO-write_bank0"=3489660929, "IO-read_bank1"=3506442240, "IO-write_bank1"=3506438145, "DA0-0_LED365"=2684354561, "DA0-1_LED385"=2685403137, "DA0-2_LED440"=2686451713, "DA0-3_LED470"=2687500289, "DA0-4_LED510"=2688548865, "DA0-5_LED550"=2689597441, "DA0-6_LED590"=2690646017, "DA0-7_LED640"=2691694593, "DA1-0_LED-R"=2701131777, "DA1-1_LED-G"=2702180353, "DA1-2_LED-B"=2703228929, "DA1-3_LED-AF"=2704277505, "DA1-4"=2705326081, "DA1-5"=2706374657, "DA1-6"=2707423233, "DA1-7"=2708471809, "DA2-Laser0"=2717908993, "DA2-Laser1"=2718957569, "DA2-Laser2"=2720006145, "DA2-Laser3"=2721054721, "DA2-Laser4"=2722103297, "Analog-read_AD0-0"=2818576384, "Analog-read-store_AD0-0"=2818572290, "IO-delay_bank0"=3489923073, "IO-delay_bank0_fromVar"=3489923075, "read_cam_clock"=3289124864, "store_cam_clock"=3289120770, "read_cam_phase"=3289190400, "store_cam_phase"=3289186306, "store_cam_phase-t"=3289190402, "Read ticks"=4026535936, "Read ticks to var"=4026535938, "Read IP"=4043313152, "Read IP into var"=4043313154, "Set IP from var"=4043309059, "Set IP from var, relative"=4043313155, "decrement_branchRel_if_equal"=4043374945, "decrement_branchRel_if_greaterequal"=4043375201, "decrement_branchRel_if_greaterequal_withTicket"=4043379297, "decrement_branchRel_if_smaller"=4043375457, "increment_branchRel_if_smaller"=4043375473, "readVar"=4060090368, "writeVar"=4060086273, "copyVar0_from_var1"=4060086275, "math_addToVariable"=4076863488, "math_addVToVariable"=4076863489, "math_subToVariable"=4076863490, "math_subVToVariable"=4076863491, "math_multToVariable"=4076863492, "math_multvToVariable"=4076863493, "math_divideToVariable"=4076863494, "math_divideVToVariable"=4076863495, "math_modToVariable"=4076863496, "math_modVToVariable"=4076863497, "logic_and"=4093640704, "logic_or"=4093640706, "logic_xor"=4093640708, "bitshift"=4093640712, "set_1Galvo"=101712113, "set_x-Galvo"=102760689, "set_y-Galvo"=103809265, "set_z-Fokus"=104857841, "set_1Galvo_position-only"=101711937, "set_x-Galvo_position-only"=102760513, "set_y-Galvo_position-only"=103809089, "set_z-Fokus_position-only"=104857665, "set_x-Galvo_position-only_ticket"=102764609, "set_y-Galvo_position-only_ticket"=103813185, "set_z-Fokus_position-only_ticket"=104861761, "set_1Galvo_relativ-only"=101712001, "set_x-Galvo_relativ-only"=102760577, "set_y-Galvo_relativ-only"=103809153, "set_z-Fokus_relativ-only"=104857729, "set_1Galvo_speed-only"=101711905, "set_x-Galvo_speed-only"=102760481, "set_y-Galvo_speed-only"=103809057, "set_z-Fokus_speed-only"=104857633, "set_1Galvo_acc-only"=101711889, "set_x-Galvo_acc-only"=102760465, "set_y-Galvo_acc-only"=103809041, "set_z-Fokus_acc-only"=104857617, "read_1Galvo_ticket"=101716032, "read_x-Galvo_ticket"=102764608, "read_y-Galvo_ticket"=103813184, "read_z-Focus_ticket"=104861760, "x-Galvo_pos_fromVar"=102760515, "y-Galvo_pos_fromVar"=103809091, "z-Focus_pos_fromVar"=104857667, "Servo0"=67108865, "Servo0-enable"=68091911, "Servo0-disable"=68091919, "Servo1"=68157441, "Servo1-enable"=69140487, "Servo1-disable"=69140495, "Servo2-enable"=70189063, "Servo2"=69206017, "Servo3-enable"=71237639, "Servo3"=70254593, "x-ssi-init"=202309639, "x-ssi-disable"=202309647, "x-ssi-Bits"=201523201, "x-ssi-Read"=201330688, "x-ssi-ReadToVar"=201326594, "x-ssi-ReadToVar-ticket"=201330690, "y-ssi-init"=203358215, "y-ssi-disable"=203358223, "y-ssi-Bits"=202571777, "y-ssi-Read"=202379264, "y-ssi-ReadToVar"=202375170, "y-ssi-ReadToVat-ticket"=202379266] ("command")
      # "orca"
      n16 = Split Number(x=w71) -> (lo(x)=w70:u16)  [unwired: 1 out]
      n17 = Split Number(x=w70) -> (lo(x)=w69:u8)  [unwired: 1 out]
      n18 = Multiply(x=w68, y=w66) -> (x*y=w67:dbl)
      n19 = Format Into String(format string="SOUR%01d:POW:LEV:IMM:AMPL %0.3f\r", w69, w67) -> (resulting string=w65:string)  [unwired: 2 in, 1 out]
      "orca string" <- w65
      n20 = call "SIAM-RS232-direkt.vi"("ReturnBytes"=u16 4, "error in (no error)"=w73, "UART: 0..3"=u8 2, "Combo Box"=w65) -> ("error out"=w72:errorcluster, "Script"=w75:T6)  [unwired: 5 in, 1 out]
    }
  }
  "error out" <- w2
  "Direct Commands" <- w5
